vi "Get VI name.vi"(11 "VI in":refnum<vi>) -> (1 "Full Vi Name":string, 2 "Plain Name":string, 3 "VI out":refnum<vi>)   [LabVIEW 2019, in "Panther Dashboard.lvlib"]
uses:
  Panther Dashboard.lvlib
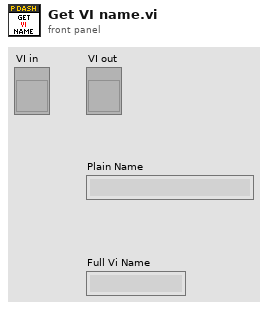
[diagram p1: front panel]
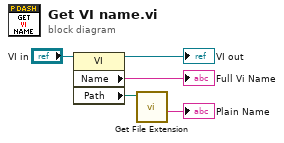
[diagram p0: block diagram]
diagram:
  n1 = property class="VI"(reference="VI in") -> (reference out=→"VI out":refnum<vi>, "Name"=→"Full Vi Name":string, "Path"=w2:path)  [unwired: 1 in, 1 out]
  n2 = call <vilib>:"Get File Extension.vi"("file"=w2) -> ("filename without extension"=→"Plain Name":string)  [unwired: 6 in, 4 out]
